vi "OpenTalonDrive.vi"   [LabVIEW 2017]
uses:
  <vilib>/Rock Robotics/WPI/SafetyOutput/WPI_SafetyOutputConfigMenu.ctl
  <vilib>/Rock Robotics/WPI/ThirdParty/Phoenix-LabVIEW/Motor Controller/Controls/CTRE_Phoenix_MotorControl_ControlMode.ctl
types:
  T1 = typedef "CTRE_Phoenix_MotorControl_ControlMode.ctl" = u16
  T2 = typedef "WPI_SafetyOutputConfigMenu.ctl" = enum16{"Enable", "Disable"}
  T3 = typedef "WPI_MotorControlDeviceRef.ctl" = cluster{"DeviceStatus":errorcluster, "Type":T4, "PWM":cluster{"PWM Channel":T5, "DeadBand":T6}, "CAN":cluster{"Device Number":u8, "SetOutput VI Ref":variant, "GetOutput VI Ref":variant, "Enable VI Ref":variant, "Disable VI Ref":variant, "Data":variant}, "Invert":bool, "DIO PWM":cluster{"PWM \"Enable\" Channel":T5, "DIOChannel":T7, "PWM Rate":dbl}}
  T4 = typedef "WPI_MotorControlType.ctl" = enum16{"PWM", "CAN", "DIO PWM"}
  T5 = typedef "FPGA_DIOPWMChannel.ctl" = enum8{"PWM 0", "PWM 1", "PWM 2", "PWM 3", "PWM 4", "PWM 5", "PWM 6", "PWM 7", "PWM 8", "PWM 9", "PWM MXP 0", "PWM MXP 1", "PWM MXP 2", "PWM MXP 3", "PWM MXP 4", "PWM MXP 5", "PWM MXP 6", "PWM MXP 7", "PWM MXP 8", "PWM MXP 9", "Invalid"}
  T6 = typedef "WPI_PWMDeadband.ctl" = cluster{"Name":string, "maxPositivePwm":i32, "minPositivePwm":i32, "centerPwm":i32, "maxNegativePwm":i32, "minNegativePwm":i32, "angularRange":u16}
  T7 = typedef "FPGA_DIOChannel.ctl" = enum8{"DIO 0", "DIO 1", "DIO 2", "DIO 3", "DIO 4", "DIO 5", "DIO 6", "DIO 7", "DIO 8", "DIO 9", "DIO MXP 0", "DIO MXP 1", "DIO MXP 2", "DIO MXP 3", "DIO MXP 4", "DIO MXP 5", "DIO MXP 6", "DIO MXP 7", "DIO MXP 8", "DIO MXP 9", "DIO MXP 10", "DIO MXP 11", "DIO MXP 12", "DIO MXP 13", "DIO MXP 14", "DIO MXP 15", "SPI Port CS1", "SPI Port CS2", "SPI Port CS3", "SPI Port MISO", "SPI Port MOSI", "Invalid"}
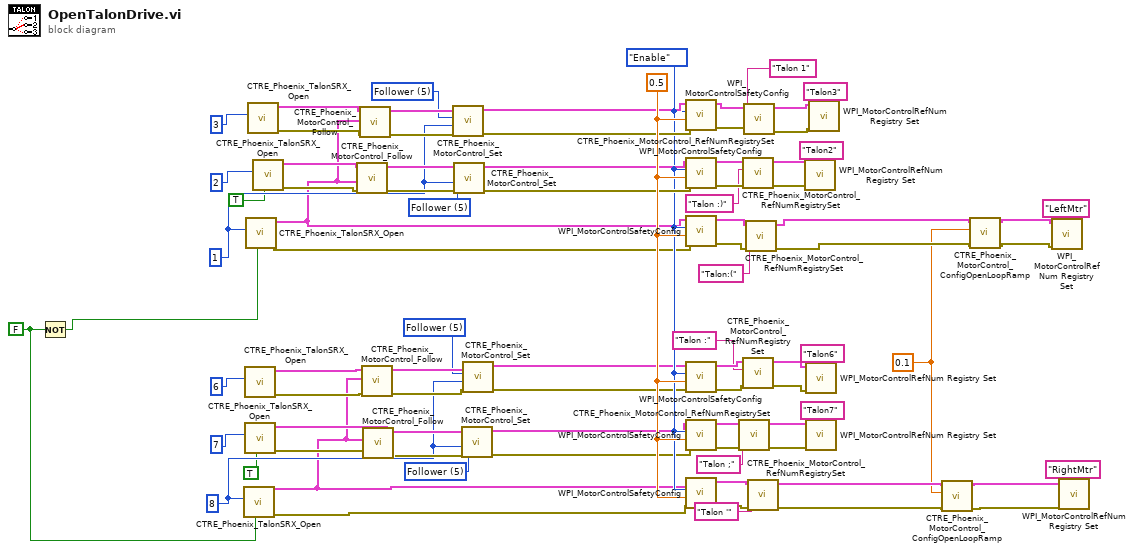
[diagram p0: block diagram]
diagram:
  w44 = T1 5 items=["PercentOutput"=0, "Position"=1, "Velocity"=2, "Current"=3, "Follower"=5, "MotionProfile"=6, "MotionMagic"=7, "MotionMagicArc"=8, "MotionProfileArc"=10, "Disabled"=15] ("Control Mode")
  w45 = T1 5 items=["PercentOutput"=0, "Position"=1, "Velocity"=2, "Current"=3, "Follower"=5, "MotionProfile"=6, "MotionMagic"=7, "MotionMagicArc"=8, "MotionProfileArc"=10, "Disabled"=15] ("Control Mode")
  w62 = T1 5 items=["PercentOutput"=0, "Position"=1, "Velocity"=2, "Current"=3, "Follower"=5, "MotionProfile"=6, "MotionMagic"=7, "MotionMagicArc"=8, "MotionProfileArc"=10, "Disabled"=15] ("Control Mode")
  w63 = T1 5 items=["PercentOutput"=0, "Position"=1, "Velocity"=2, "Current"=3, "Follower"=5, "MotionProfile"=6, "MotionMagic"=7, "MotionMagicArc"=8, "MotionProfileArc"=10, "Disabled"=15] ("Control Mode")
  w5 = 0.1 ("Throttle Ramp Rate (percent/s)")
  w59 = FALSE
  w54 = WPI_SafetyOutputConfigMenu."Enable" ("mode")
  w42 = u8 8 ("Device Number")
  w83 = 0.5 ("timeout (s)")
  w61 = u8 1 ("Device Number")
  n1 = Not(x=w59) -> (.not. x?=w76:bool)
  n2 = call <vilib>:"CTRE_Phoenix_TalonSRX_Open.vi"("Invert"=w59, "Device Number"=w42) -> ("error out"=w4:errorcluster, "CAN Talon SRX Ref"=w3:T3)  [unwired: 8 in]
  n3 = call <vilib>:"CTRE_Phoenix_TalonSRX_Open.vi"("Device Number"=u8 6) -> ("error out"=w56:errorcluster, "CAN Talon SRX Ref"=w57:T3)  [unwired: 9 in]
  n4 = call <vilib>:"CTRE_Phoenix_TalonSRX_Open.vi"("Invert"=TRUE, "Device Number"=u8 7) -> ("error out"=w55:errorcluster, "CAN Talon SRX Ref"=w58:T3)  [unwired: 8 in]
  n5 = call <vilib>:"CTRE_Phoenix_TalonSRX_Open.vi"("Invert"=w76, "Device Number"=w61) -> ("error out"=w2:errorcluster, "CAN Talon SRX Ref"=w1:T3)  [unwired: 8 in]
  n6 = call <vilib>:"CTRE_Phoenix_TalonSRX_Open.vi"("Device Number"=u8 3) -> ("error out"=w75:errorcluster, "CAN Talon SRX Ref"=w73:T3)  [unwired: 9 in]
  n7 = call <vilib>:"CTRE_Phoenix_TalonSRX_Open.vi"("Invert"=TRUE, "Device Number"=u8 2) -> ("error out"=w74:errorcluster, "CAN Talon SRX Ref"=w72:T3)  [unwired: 8 in]
  n8 = call <vilib>:"CTRE_Phoenix_MotorControl_Follow.vi"("error in (no error)"=w74, "Master Controller to Follow"=w1, "PhoenixMotorControlDevRef"=w72) -> ("error out"=w67:errorcluster, "PhoenixMotorControlDevRef"=w65:T3)  [unwired: 7 in]
  n9 = call <vilib>:"CTRE_Phoenix_MotorControl_Follow.vi"("error in (no error)"=w75, "Master Controller to Follow"=w1, "PhoenixMotorControlDevRef"=w73) -> ("error out"=w69:errorcluster, "PhoenixMotorControlDevRef"=w71:T3)  [unwired: 7 in]
  n10 = call <vilib>:"CTRE_Phoenix_MotorControl_Follow.vi"("error in (no error)"=w56, "Master Controller to Follow"=w3, "PhoenixMotorControlDevRef"=w57) -> ("error out"=w47:errorcluster, "PhoenixMotorControlDevRef"=w49:T3)  [unwired: 7 in]
  n11 = call <vilib>:"CTRE_Phoenix_MotorControl_Follow.vi"("error in (no error)"=w55, "Master Controller to Follow"=w3, "PhoenixMotorControlDevRef"=w58) -> ("error out"=w53:errorcluster, "PhoenixMotorControlDevRef"=w51:T3)  [unwired: 7 in]
  n12 = call <vilib>:"CTRE_Phoenix_MotorControl_Set.vi"("error in (no error)"=w69, "Output"=w61, "Control Mode"=w62, "PhoenixMotorControlDevRef"=w71) -> ("error out"=w68:errorcluster, "PhoenixMotorControlDevRef"=w70:T3)  [unwired: 6 in]
  n13 = call <vilib>:"CTRE_Phoenix_MotorControl_Set.vi"("error in (no error)"=w67, "Output"=w61, "Control Mode"=w63, "PhoenixMotorControlDevRef"=w65) -> ("error out"=w66:errorcluster, "PhoenixMotorControlDevRef"=w64:T3)  [unwired: 6 in]
  n14 = call <vilib>:"CTRE_Phoenix_MotorControl_Set.vi"("error in (no error)"=w53, "Output"=w42, "Control Mode"=w44, "PhoenixMotorControlDevRef"=w51) -> ("error out"=w52:errorcluster, "PhoenixMotorControlDevRef"=w50:T3)  [unwired: 6 in]
  n15 = call <vilib>:"CTRE_Phoenix_MotorControl_Set.vi"("error in (no error)"=w47, "Output"=w42, "Control Mode"=w45, "PhoenixMotorControlDevRef"=w49) -> ("error out"=w46:errorcluster, "PhoenixMotorControlDevRef"=w48:T3)  [unwired: 6 in]
  n16 = call <vilib>:"WPI_MotorControlSafetyConfig.vi"("error in (no error)"=w68, "timeout (s)"=w83, "mode"=w54, "MotorControlDevRef"=w70) -> ("error out"=w41:errorcluster, "MotorControlDevRef"=w39:T3)  [unwired: 6 in]
  n17 = call <vilib>:"WPI_MotorControlSafetyConfig.vi"("error in (no error)"=w66, "timeout (s)"=w83, "mode"=w54, "MotorControlDevRef"=w64) -> ("error out"=w34:errorcluster, "MotorControlDevRef"=w32:T3)  [unwired: 6 in]
  n18 = call <vilib>:"WPI_MotorControlSafetyConfig.vi"("error in (no error)"=w2, "timeout (s)"=w83, "mode"=w54, "MotorControlDevRef"=w1) -> ("error out"=w30:errorcluster, "MotorControlDevRef"=w29:T3)  [unwired: 6 in]
  n19 = call <vilib>:"WPI_MotorControlSafetyConfig.vi"("error in (no error)"=w46, "timeout (s)"=w83, "mode"=w54, "MotorControlDevRef"=w48) -> ("error out"=w25:errorcluster, "MotorControlDevRef"=w19:T3)  [unwired: 6 in]
  n20 = call <vilib>:"WPI_MotorControlSafetyConfig.vi"("error in (no error)"=w52, "timeout (s)"=w83, "mode"=w54, "MotorControlDevRef"=w50) -> ("error out"=w28:errorcluster, "MotorControlDevRef"=w21:T3)  [unwired: 6 in]
  n21 = call <vilib>:"WPI_MotorControlSafetyConfig.vi"("error in (no error)"=w4, "timeout (s)"=w83, "mode"=w54, "MotorControlDevRef"=w3) -> ("error out"=w27:errorcluster, "MotorControlDevRef"=w17:T3)  [unwired: 6 in]
  n22 = call <vilib>:"CTRE_Phoenix_MotorControl_RefNumRegistrySet.vi"("error in (no error)"=w28, "refnum name"="Talon ;", "PhoenixMotorControlDevRef"=w21) -> ("error out"=w26:errorcluster, "PhoenixMotorControlDevRef"=w20:T3)  [unwired: 7 in]
  n23 = call <vilib>:"CTRE_Phoenix_MotorControl_RefNumRegistrySet.vi"("error in (no error)"=w34, "refnum name"="Talon :)", "PhoenixMotorControlDevRef"=w32) -> ("error out"=w33:errorcluster, "PhoenixMotorControlDevRef"=w31:T3)  [unwired: 7 in]
  n24 = call <vilib>:"CTRE_Phoenix_MotorControl_RefNumRegistrySet.vi"("error in (no error)"=w25, "refnum name"="Talon :", "PhoenixMotorControlDevRef"=w19) -> ("error out"=w24:errorcluster, "PhoenixMotorControlDevRef"=w18:T3)  [unwired: 7 in]
  n25 = call <vilib>:"CTRE_Phoenix_MotorControl_RefNumRegistrySet.vi"("error in (no error)"=w41, "refnum name"="Talon 1", "PhoenixMotorControlDevRef"=w39) -> ("error out"=w40:errorcluster, "PhoenixMotorControlDevRef"=w38:T3)  [unwired: 7 in]
  n26 = call <vilib>:"CTRE_Phoenix_MotorControl_RefNumRegistrySet.vi"("error in (no error)"=w30, "refnum name"="Talon:(", "PhoenixMotorControlDevRef"=w29) -> ("error out"=w10:errorcluster, "PhoenixMotorControlDevRef"=w13:T3)  [unwired: 7 in]
  n27 = call <vilib>:"CTRE_Phoenix_MotorControl_RefNumRegistrySet.vi"("error in (no error)"=w27, "refnum name"="Talon '", "PhoenixMotorControlDevRef"=w17) -> ("error out"=w7:errorcluster, "PhoenixMotorControlDevRef"=w6:T3)  [unwired: 7 in]
  n28 = call <vilib>:"WPI_MotorControlRefNum Registry Set.vi"("error in (no error)"=w33, "refnum name"="Talon2", "MotorControlDevRef"=w31) -> ()  [unwired: 7 in, 2 out]
  n29 = call <vilib>:"WPI_MotorControlRefNum Registry Set.vi"("error in (no error)"=w24, "refnum name"="Talon6", "MotorControlDevRef"=w18) -> ()  [unwired: 7 in, 2 out]
  n30 = call <vilib>:"WPI_MotorControlRefNum Registry Set.vi"("error in (no error)"=w26, "refnum name"="Talon7", "MotorControlDevRef"=w20) -> ()  [unwired: 7 in, 2 out]
  n31 = call <vilib>:"WPI_MotorControlRefNum Registry Set.vi"("error in (no error)"=w40, "refnum name"="Talon3", "MotorControlDevRef"=w38) -> ()  [unwired: 7 in, 2 out]
  n32 = call <vilib>:"CTRE_Phoenix_MotorControl_ConfigOpenLoopRamp.vi"("error in (no error)"=w7, "secondsFromNeutralToFull"=w5, "PhoenixMotorControlDevRef"=w6) -> ("error out"=w8:errorcluster, "PhoenixMotorControlDevRef"=w9:T3)  [unwired: 7 in]
  n33 = call <vilib>:"CTRE_Phoenix_MotorControl_ConfigOpenLoopRamp.vi"("error in (no error)"=w10, "secondsFromNeutralToFull"=w5, "PhoenixMotorControlDevRef"=w13) -> ("error out"=w11:errorcluster, "PhoenixMotorControlDevRef"=w12:T3)  [unwired: 7 in]
  n34 = call <vilib>:"WPI_MotorControlRefNum Registry Set.vi"("error in (no error)"=w11, "refnum name"="LeftMtr" ("Ref Name 1"), "MotorControlDevRef"=w12) -> ()  [unwired: 7 in, 2 out]
  n35 = call <vilib>:"WPI_MotorControlRefNum Registry Set.vi"("error in (no error)"=w8, "refnum name"="RightMtr" ("Ref Name 2"), "MotorControlDevRef"=w9) -> ()  [unwired: 7 in, 2 out]
